vi "GetErrorMessage.vi"(10 "error in (no error)":errorcluster) -> (2 "Error Message":string)   [LabVIEW 2017, in "Constraint.lvlib" / "ErrorMessageContains.lvclass"]
uses:
  ErrorMessageContains.lvclass
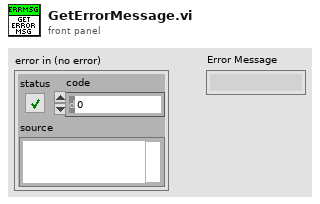
[diagram p1: front panel]
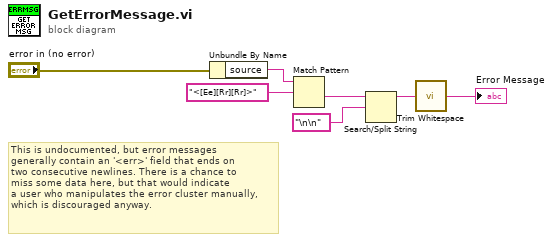
[diagram p0: block diagram]
diagram:
  # "This is undocumented, but error messages\ngenerally contain an '<err>' field that ends on\ntwo consecutive newlines. There is a chance to\nmiss some data here, but that would indicate\na user who manipulates the error cluster manually,\nwhich is discouraged anyway."
  n1 = Unbundle By Name("error in (no error)") -> ("source"=w6:string)
  n2 = Match Pattern(string=w6, regular expression="<[Ee][Rr][Rr]>") -> (after substring=w5:string)  [unwired: 1 in, 3 out]
  n3 = Search/Split String(string=w5, search string/char (-)="\n\n") -> (substring before match=w3:string)  [unwired: 1 in, 2 out]
  n4 = call <vilib>:"Trim Whitespace.vi"("string"=w3) -> ("trimmed string"=→"Error Message":string)  [unwired: 1 in]
